vi "(FULLTASK) - Complete full auto.vi"() -> ()   [LabVIEW 2016, in "testrobot.lvrbt"]
uses:
  testrobot.lvrbt
  <vilib>/NXT/Block Support/NXT_InputPort.ctl
  <vilib>/NXT/Subs/LVHSConnector.ctl
  <vilib>/NXT/LegoClasses/BrickReference/BrickReference.lvclass
  <vilib>/NXT/Block Support/NXT_OutputPort.ctl
panel:
  out "Left 6":sgl
  out "Right 6":sgl
  out "forward 3":bool
  out "Right 5":bool
  out "Left 5":bool
  out "both positve 3":bool
  out "only right 3":bool
  out "both negative 3":bool
  in  "right light 3":T1=3 items=["Port 1", "Port 2", "Port 3", "Port 4"]
  in  "left light 3":T1 items=["Port 1", "Port 2", "Port 3", "Port 4"]
  out "NXT/EV3 2":T2
  out "Left 4":sgl
  out "Right 4":sgl
  out "forward 2":bool
  out "Right 3":bool
  out "Left 3":bool
  out "both positve 2":bool
  out "only right 2":bool
  out "both negative 2":bool
  in  "right light 2":T1 items=["Port 1", "Port 2", "Port 3", "Port 4"]
  in  "left light 2":T1 items=["Port 1", "Port 2", "Port 3", "Port 4"]
  in  "ultra":T1 items=["Port 1", "Port 2", "Port 3", "Port 4"]
  out "Distance":dbl
  in  "NXT/EV3":T2
  out "Left 2":sgl
  out "Right 2":sgl
  out "forward":bool
  out "Right":bool
  out "Left":bool
  out "both positve":bool
  out "only right":bool
  out "both negative":bool
  in  "right light":T1=3 items=["Port 1", "Port 2", "Port 3", "Port 4"]
  in  "left light":T1 items=["Port 1", "Port 2", "Port 3", "Port 4"]
  out "Scaled dif":dbl
  in  "Force":T1=1 items=["Port 1", "Port 2", "Port 3", "Port 4"]
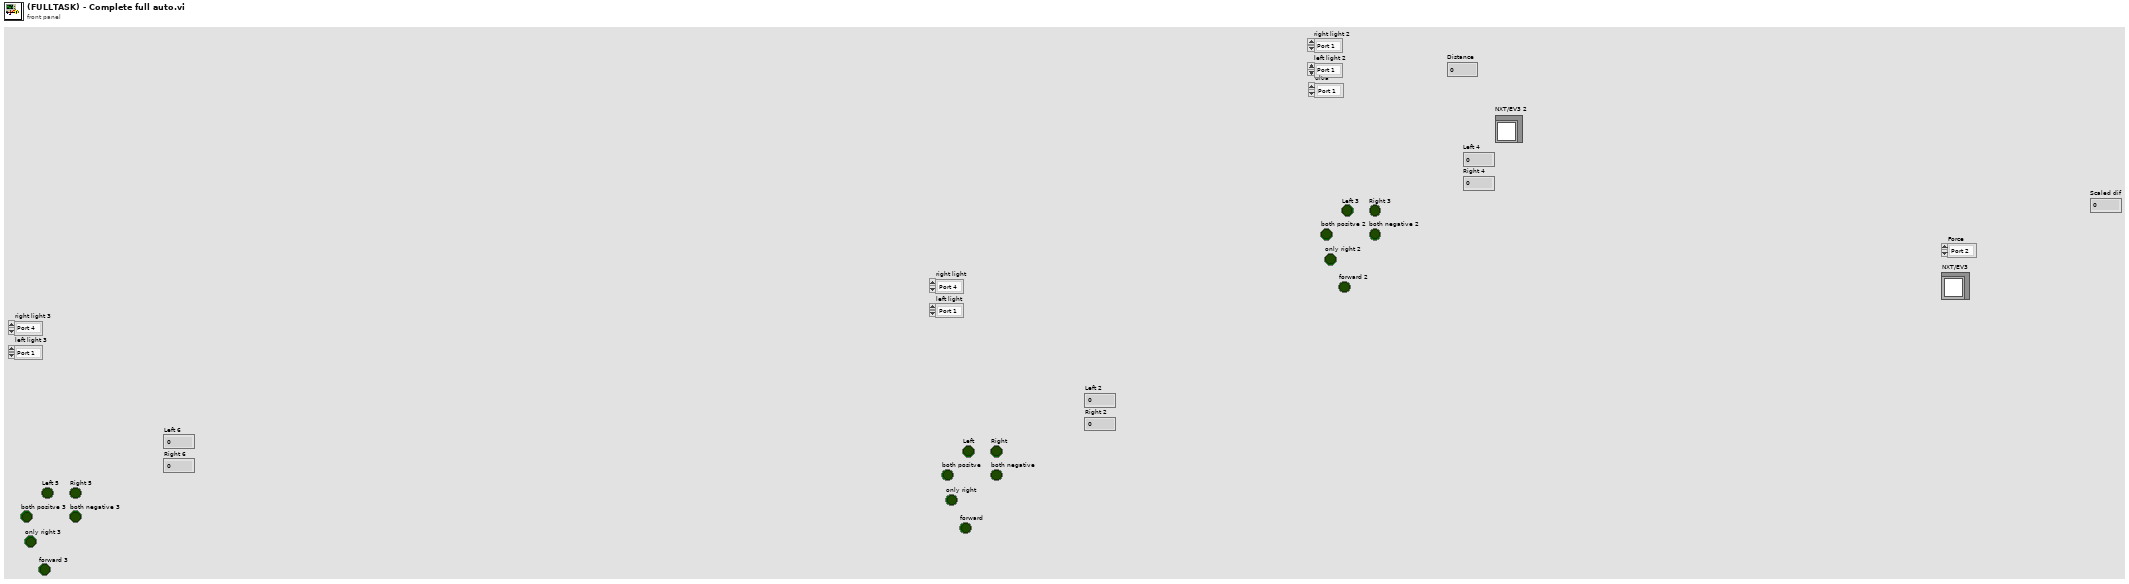
[diagram p1: front panel]
types:
  T1 = typedef "NXT_InputPort.ctl" = u32
  T2 = typedef "LVHSConnector.ctl" = refnum<class "BrickReference.lvclass">
  T3 = typedef "NXT_OutputPort.ctl" = u8
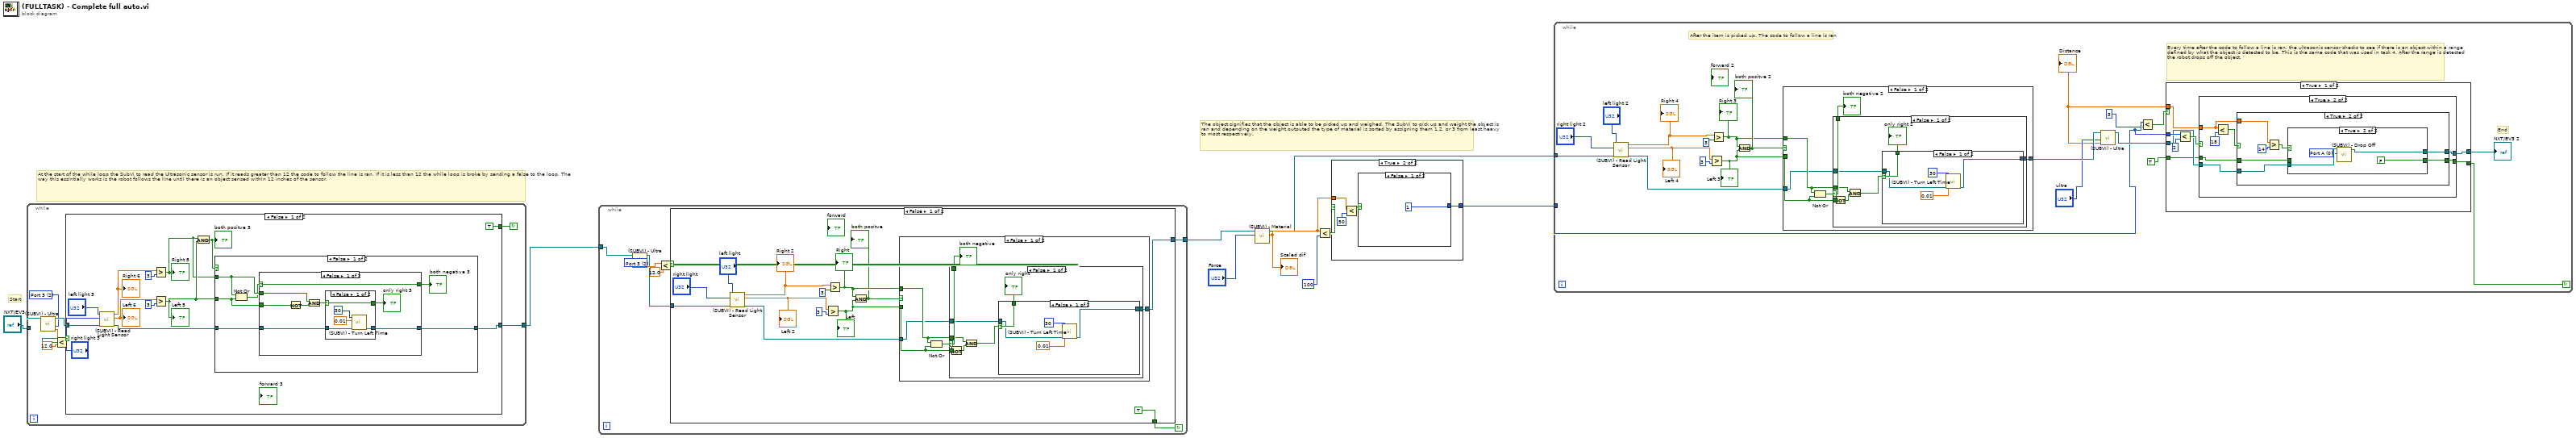
[diagram p0: block diagram]
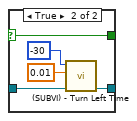
[diagram p2: hidden frame]
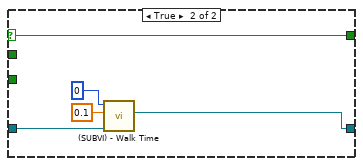
[diagram p3: hidden frame]
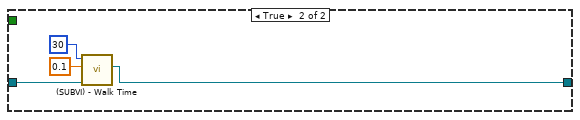
[diagram p4: hidden frame]
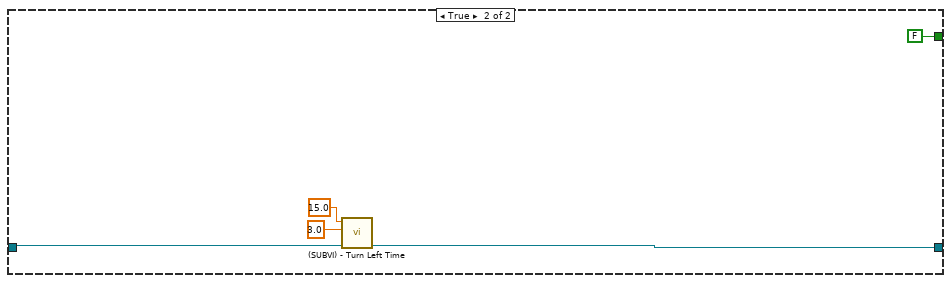
[diagram p5: hidden frame]
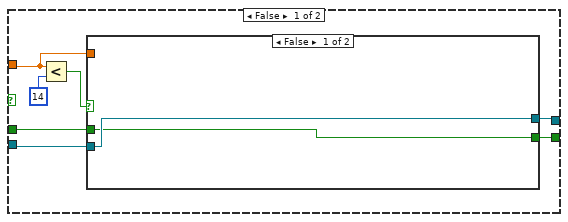
[diagram p6: hidden frame]
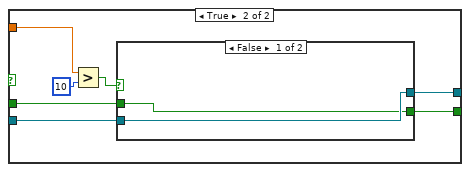
[diagram p7: hidden frame]
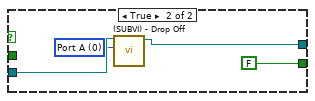
[diagram p8: hidden frame]
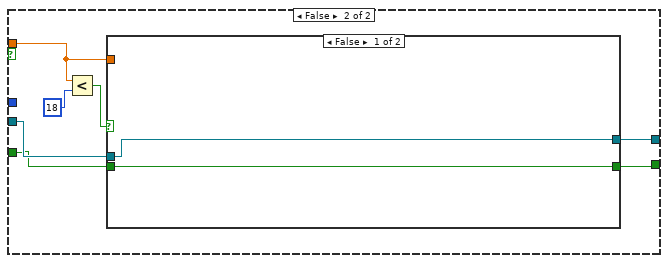
[diagram p11: hidden frame]
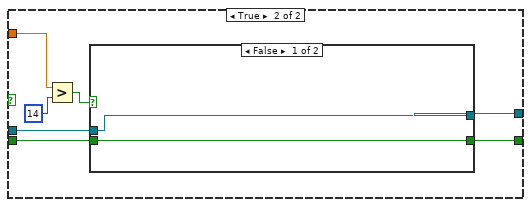
[diagram p12: hidden frame]
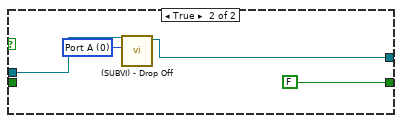
[diagram p13: hidden frame]
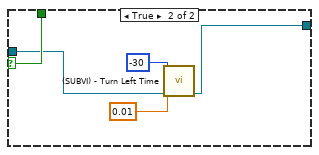
[diagram p14: hidden frame]
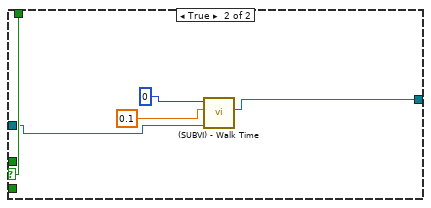
[diagram p15: hidden frame]
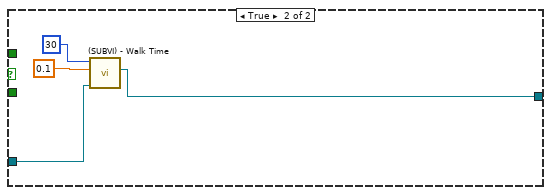
[diagram p16: hidden frame]
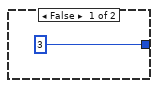
[diagram p17: hidden frame]
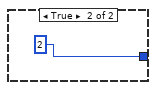
[diagram p18: hidden frame]
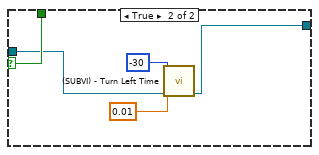
[diagram p19: hidden frame]
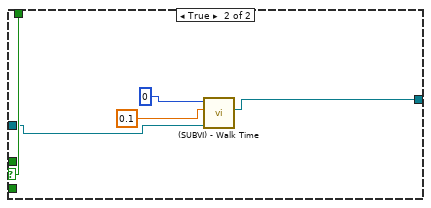
[diagram p20: hidden frame]
diagram:
  # "The object signifies that the object is able to be picked up and weighed. The SubVi to pick up and weight the object is ran and depending on the weight outputed the type of material is sorted by assigning them 1,2, or 3 from least heavy to most respectively."
  # "At the start of the while loop the SubVi to read the Ultrasonic sensor is run. If it reads greater than 12 the code to follow the line is ran. If it is less than 12 the while loop is broke by sending a false to the loop. The way this essintially works is the robot follows the line until there is an object sensed within 12 inches of the sensor."
  # "Start"
  n1 = while {
    tunnel: [w12] -> w1
    tunnel: "NXT/EV3" -> [w10]
    stop <- w14 continue-if-true
    w11 = T1 2 items=["Port 1", "Port 2", "Port 3", "Port 4"] ("Port (Port 1)")
    n2 = call "(SUBVI) - Ultra.vi"("Port (Port 1)"=w11, "NXT/EV3"=w10) -> ("Inches"=w17:sgl, "NXT/EV3 2"=w13:T2)  [unwired: 8 in]
    n3 = Less?(x=w17, y=sgl 12.0 ("x")) -> (x < y?=w15:bool)
    n4 = case shown="False" w15 {
      tunnel: [TRUE FALSE] -> w14
      tunnel: w13 -> [w20 w67]
      tunnel: [w19 w66] -> w12
      frame False {
        n5 = call "(SUBVI) - Read Light Sensor.vi"("NXT/EV3"=w20, "Port (Port 1) 2"="right light 3", "Port (Port 1)"="left light 3") -> ("NXT/EV3 2"=w26:T2, "Scaled Value 2"=w23:sgl, "Scaled Value"=w24:sgl)  [unwired: 6 in]
        "Left 6" <- w23
        "Right 6" <- w24
        n6 = Greater?(x=w24, y=3) -> (0:w27:bool)
        "Right 5" <- w27
        n7 = Greater?(x=w23, y=3) -> (0:w28:bool)
        "Left 5" <- w28
        n8 = And(x=w27, y=w28) -> (x .and. y?=w25:bool)
        "both positve 3" <- w25
        n9 = case shown="False" w25 {
          tunnel: w26 -> [w32 w61]
          tunnel: [w31 w60] -> w19
          tunnel: w27 -> [w35 _]
          tunnel: w28 -> [w34 _]
          frame False {
            n10 = Not Or(1:w34, 2:w35) -> (0:w33:bool)
            n11 = case shown="False" w33 {
              selector: w33 -> [w44 w59]
              tunnel: [w44 w59] -> w36
              tunnel: w35 -> [w42 _]
              tunnel: w34 -> [w40 _]
              tunnel: w32 -> [w38 w56]
              tunnel: [w37 w55] -> w31
              frame False {
                n12 = Not(x=w40) -> (.not. x?=w41:bool)
                n13 = And(x=w42, y=w41) -> (x .and. y?=w43:bool)
                n14 = case shown="False" w43 {
                  selector: w43 -> [w49 w54]
                  tunnel: [w49 w54] -> w39
                  tunnel: w38 -> [w46 w51]
                  tunnel: [w45 w50] -> w37
                  frame False {
                    n15 = call "(SUBVI) - Turn Left Time.vi"("NXT/EV3"=w46, "Time walking"=0.01, "Walk Speed"=30) -> ("NXT/EV3 2"=w45:T2)  [unwired: 8 in]
                  }
                  frame True {
                    n16 = call "(SUBVI) - Turn Left Time.vi"("NXT/EV3"=w51, "Time walking"=0.01, "Walk Speed"=-30) -> ("NXT/EV3 2"=w50:T2)  [unwired: 8 in]
                  }
                }
                "only right 3" <- w39
              }
              frame True {
                n17 = call "(SUBVI) - Walk Time.vi"("NXT/EV3"=w56, "Time walking"=0.1, "Walk Speed"=0) -> ("NXT/EV3 2"=w55:T2)  [unwired: 8 in]
              }
            }
            "both negative 3" <- w36
          }
          frame True {
            n18 = call "(SUBVI) - Walk Time.vi"("NXT/EV3"=w61, "Time walking"=0.1, "Walk Speed"=30) -> ("NXT/EV3 2"=w60:T2)  [unwired: 8 in]
          }
        }
      }
      frame True {
        n19 = call "(SUBVI) - Turn Left Time.vi"("NXT/EV3"=w67, "Time walking"=3.0, "Walk Speed"=15.0) -> ("NXT/EV3 2"=w66:T2)  [unwired: 8 in]
      }
    }
  }
  n20 = while {
    tunnel: [w71] -> w8
    tunnel: w1 -> [w69]
    stop <- w73 continue-if-true
    w70 = T1 2 items=["Port 1", "Port 2", "Port 3", "Port 4"] ("Port (Port 1)")
    n21 = call "(SUBVI) - Ultra.vi"("Port (Port 1)"=w70, "NXT/EV3"=w69) -> ("Inches"=w76:sgl, "NXT/EV3 2"=w72:T2)  [unwired: 8 in]
    n22 = Less?(x=w76, y=sgl 12.0 ("x")) -> (x < y?=w74:bool)
    n23 = case shown="False" w74 {
      tunnel: [TRUE FALSE] -> w73
      tunnel: w72 -> [w79 w123]
      tunnel: [w78 w123] -> w71
      frame False {
        n24 = call "(SUBVI) - Read Light Sensor.vi"("NXT/EV3"=w79, "Port (Port 1) 2"="right light", "Port (Port 1)"="left light") -> ("NXT/EV3 2"=w85:T2, "Scaled Value 2"=w82:sgl, "Scaled Value"=w83:sgl)  [unwired: 6 in]
        "Left 2" <- w82
        "Right 2" <- w83
        n25 = Greater?(x=w82, y=3) -> (0:w87:bool)
        "Left" <- w87
        n26 = Greater?(x=w83, y=3) -> (0:w86:bool)
        "Right" <- w86
        n27 = And(x=w86, y=w87) -> (x .and. y?=w84:bool)
        "both positve" <- w84
        n28 = case shown="False" w84 {
          tunnel: w85 -> [w91 w120]
          tunnel: [w90 w119] -> w78
          tunnel: w86 -> [w94 _]
          tunnel: w87 -> [w93 _]
          frame False {
            n29 = Not Or(1:w93, 2:w94) -> (0:w92:bool)
            n30 = case shown="False" w92 {
              selector: w92 -> [w103 w118]
              tunnel: [w103 w118] -> w95
              tunnel: w94 -> [w101 _]
              tunnel: w93 -> [w99 _]
              tunnel: w91 -> [w97 w115]
              tunnel: [w96 w114] -> w90
              frame False {
                n31 = Not(x=w99) -> (.not. x?=w100:bool)
                n32 = And(x=w101, y=w100) -> (x .and. y?=w102:bool)
                n33 = case shown="False" w102 {
                  selector: w102 -> [w108 w113]
                  tunnel: [w108 w113] -> w98
                  tunnel: w97 -> [w105 w110]
                  tunnel: [w104 w109] -> w96
                  frame False {
                    n34 = call "(SUBVI) - Turn Left Time.vi"("NXT/EV3"=w105, "Time walking"=0.01, "Walk Speed"=30) -> ("NXT/EV3 2"=w104:T2)  [unwired: 8 in]
                  }
                  frame True {
                    n35 = call "(SUBVI) - Turn Left Time.vi"("NXT/EV3"=w110, "Time walking"=0.01, "Walk Speed"=-30) -> ("NXT/EV3 2"=w109:T2)  [unwired: 8 in]
                  }
                }
                "only right" <- w98
              }
              frame True {
                n36 = call "(SUBVI) - Walk Time.vi"("NXT/EV3"=w115, "Time walking"=0.1, "Walk Speed"=0) -> ("NXT/EV3 2"=w114:T2)  [unwired: 8 in]
              }
            }
            "both negative" <- w95
          }
          frame True {
            n37 = call "(SUBVI) - Walk Time.vi"("NXT/EV3"=w120, "Time walking"=0.1, "Walk Speed"=30) -> ("NXT/EV3 2"=w119:T2)  [unwired: 8 in]
          }
        }
      }
      frame True {
      }
    }
  }
  n38 = call "(SUBVI) - Material.vi"("Port (Port 1)"="Force", "NXT/EV3"=w8) -> ("Scaled dif"=w5:dbl, "NXT/EV3 2"=w3:T2)  [unwired: 8 in]
  "Scaled dif" <- w5
  n39 = Less?(x=w5, y=100) -> (x < y?=w7:bool)
  n40 = case shown="True" w7 {
    tunnel: w5 -> [_ w129]
    tunnel: [3 w126] -> w4
    frame False {
    }
    frame True {
      n41 = Less?(x=w129, y=50) -> (x < y?=w128:bool)
      n42 = case shown="False" w128 {
        tunnel: [1 2] -> w126
        frame False {
        }
        frame True {
        }
      }
    }
  }
  n43 = while {
    tunnel: w3 -> [w141]
    tunnel: w4 -> [w137]
    stop <- w133 continue-if-true
    # "End"
    # "Every time after the code to follow a line is ran, the ultrasonic sensor checks to see if there is an object within a range defined by what the object is detected to be. This is the same code that was used in task 4. After the range is detected the robot drops off the object."
    # "After the item is picked up. The code to follow a line is ran"
    n44 = call "(SUBVI) - Read Light Sensor.vi"("NXT/EV3"=w141, "Port (Port 1) 2"="right light 2", "Port (Port 1)"="left light 2") -> ("NXT/EV3 2"=w147:T2, "Scaled Value 2"=w150:sgl, "Scaled Value"=w149:sgl)  [unwired: 6 in]
    "Left 4" <- w150
    "Right 4" <- w149
    n45 = Greater?(x=w150, y=3) -> (0:w145:bool)
    "Left 3" <- w145
    n46 = Greater?(x=w149, y=3) -> (0:w146:bool)
    "Right 3" <- w146
    n47 = And(x=w146, y=w145) -> (x .and. y?=w148:bool)
    "both positve 2" <- w148
    n48 = case shown="False" w148 {
      tunnel: w147 -> [w228 w257]
      tunnel: [w227 w256] -> w142
      tunnel: w146 -> [w231 _]
      tunnel: w145 -> [w230 _]
      frame False {
        n49 = Not Or(1:w230, 2:w231) -> (0:w229:bool)
        n50 = case shown="False" w229 {
          selector: w229 -> [w240 w255]
          tunnel: [w240 w255] -> w232
          tunnel: w231 -> [w238 _]
          tunnel: w230 -> [w236 _]
          tunnel: w228 -> [w234 w252]
          tunnel: [w233 w251] -> w227
          frame False {
            n51 = Not(x=w236) -> (.not. x?=w237:bool)
            n52 = And(x=w238, y=w237) -> (x .and. y?=w239:bool)
            n53 = case shown="False" w239 {
              selector: w239 -> [w245 w250]
              tunnel: [w245 w250] -> w235
              tunnel: w234 -> [w242 w247]
              tunnel: [w241 w246] -> w233
              frame False {
                n54 = call "(SUBVI) - Turn Left Time.vi"("NXT/EV3"=w242, "Time walking"=0.01, "Walk Speed"=30) -> ("NXT/EV3 2"=w241:T2)  [unwired: 8 in]
              }
              frame True {
                n55 = call "(SUBVI) - Turn Left Time.vi"("NXT/EV3"=w247, "Time walking"=0.01, "Walk Speed"=-30) -> ("NXT/EV3 2"=w246:T2)  [unwired: 8 in]
              }
            }
            "only right 2" <- w235
          }
          frame True {
            n56 = call "(SUBVI) - Walk Time.vi"("NXT/EV3"=w252, "Time walking"=0.1, "Walk Speed"=0) -> ("NXT/EV3 2"=w251:T2)  [unwired: 8 in]
          }
        }
        "both negative 2" <- w232
      }
      frame True {
        n57 = call "(SUBVI) - Walk Time.vi"("NXT/EV3"=w257, "Time walking"=0.1, "Walk Speed"=30) -> ("NXT/EV3 2"=w256:T2)  [unwired: 8 in]
      }
    }
    n58 = call "(SUBVI) - Ultra.vi"("Port (Port 1)"="ultra", "NXT/EV3"=w142) -> ("Inches"=w135:sgl, "NXT/EV3 2"=w140:T2)  [unwired: 8 in]
    "Distance" <- w135
    n59 = Less?(x=w137, y=3) -> (x < y?=w138:bool)
    n60 = case shown="True" w138 {
      tunnel: w140 -> [w156 w208]
      tunnel: w137 -> [w160 _]
      tunnel: w135 -> [w157 w209]
      tunnel: [w155 w207] -> w134
      tunnel: [w154 w206] -> w133
      tunnel: TRUE -> [w153 w205]
      frame True {
        n61 = Less?(x=w160, y=2) -> (x < y?=w158:bool)
        n62 = case shown="True" w158 {
          tunnel: w157 -> [w164 w187]
          tunnel: w156 -> [w165 w186]
          tunnel: [w163 w185] -> w155
          tunnel: [w162 w184] -> w154
          tunnel: w153 -> [w161 w183]
          frame False {
            n63 = Less?(x=w164, y=14) -> (x < y?=w167:bool)
            n64 = case shown="False" w167 {
              tunnel: w164 -> [_ w175]
              tunnel: w165 -> [w169 w173]
              tunnel: [w169 w172] -> w163
              tunnel: [w168 w171] -> w162
              tunnel: w161 -> [w168 w170]
              frame False {
              }
              frame True {
                n65 = Greater?(x=w175, y=10) -> (0:w174:bool)
                n66 = case shown="False" w174 {
                  tunnel: w173 -> [w178 w182]
                  tunnel: [w178 w181] -> w172
                  tunnel: [w177 FALSE] -> w171
                  tunnel: w170 -> [w177 _]
                  frame False {
                  }
                  frame True {
                    w180 = T3 0 items=["Port A", "Port B", "Port C", "Port D"] ("Motors")
                    n67 = call "(SUBVI) - Drop Off.vi"("Motors"=w180, "NXT/EV3"=w182) -> ("NXT/EV3 2"=w181:T2)  [unwired: 9 in]
                  }
                }
              }
            }
          }
          frame True {
            n68 = Less?(x=w187, y=18) -> (x < y?=w188:bool)
            n69 = case shown="True" w188 {
              tunnel: w187 -> [_ w197]
              tunnel: w186 -> [w191 w195]
              tunnel: [w191 w194] -> w185
              tunnel: [w190 w193] -> w184
              tunnel: w183 -> [w190 w192]
              frame False {
              }
              frame True {
                n70 = Greater?(x=w197, y=14) -> (0:w196:bool)
                n71 = case shown="True" w196 {
                  tunnel: w195 -> [w200 w204]
                  tunnel: [w200 w203] -> w194
                  tunnel: [w199 FALSE] -> w193
                  tunnel: w192 -> [w199 _]
                  frame False {
                  }
                  frame True {
                    w202 = T3 0 items=["Port A", "Port B", "Port C", "Port D"] ("Motors")
                    n72 = call "(SUBVI) - Drop Off.vi"("Motors"=w202, "NXT/EV3"=w204) -> ("NXT/EV3 2"=w203:T2)  [unwired: 9 in]
                  }
                }
              }
            }
          }
        }
      }
      frame False {
        n73 = Less?(x=w209, y=18) -> (x < y?=w210:bool)
        n74 = case shown="False" w210 {
          tunnel: w209 -> [_ w220]
          tunnel: w208 -> [w213 w217]
          tunnel: [w213 w216] -> w207
          tunnel: [w212 w215] -> w206
          tunnel: w205 -> [w212 w214]
          frame False {
          }
          frame True {
            n75 = Greater?(x=w220, y=14) -> (0:w218:bool)
            n76 = case shown="False" w218 {
              tunnel: w217 -> [w222 w226]
              tunnel: [w222 w225] -> w216
              tunnel: [w221 FALSE] -> w215
              tunnel: w214 -> [w221 _]
              frame False {
              }
              frame True {
                w224 = T3 0 items=["Port A", "Port B", "Port C", "Port D"] ("Motors")
                n77 = call "(SUBVI) - Drop Off.vi"("Motors"=w224, "NXT/EV3"=w226) -> ("NXT/EV3 2"=w225:T2)  [unwired: 9 in]
              }
            }
          }
        }
      }
    }
    "NXT/EV3 2" <- w134
  }
